vi "Get Display String.vi"(11 "Int GTLT in":refnum<class "Int GTLT.lvclass">) -> (2 "Display String":string)   [LabVIEW 2018, in "Int GTLT.lvclass"]
uses:
  Int GTLT.lvclass
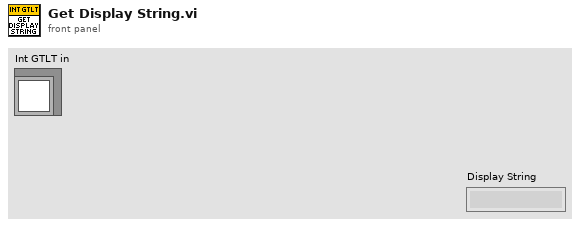
[diagram p1: front panel]
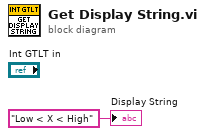
[diagram p0: block diagram]
diagram:
  "Display String" <- "Low < X < High" ("Display String")
